vi "Set Cell Colors.vi"(0 "MulticolumnListbox in":refnum<vi>, 7 "Columns":T1[](array[typedef]), 9 "Table Items":string[][](array[string]), 11 "error in (no error)":errorcluster) -> (4 "MulticolumnListbox out":refnum<vi>, 15 "error out":errorcluster)   [LabVIEW 2015, in "KTable.xctl"]
uses:
  KTable.xctl
  ColumnSpec.ctl
  ColumnType.ctl
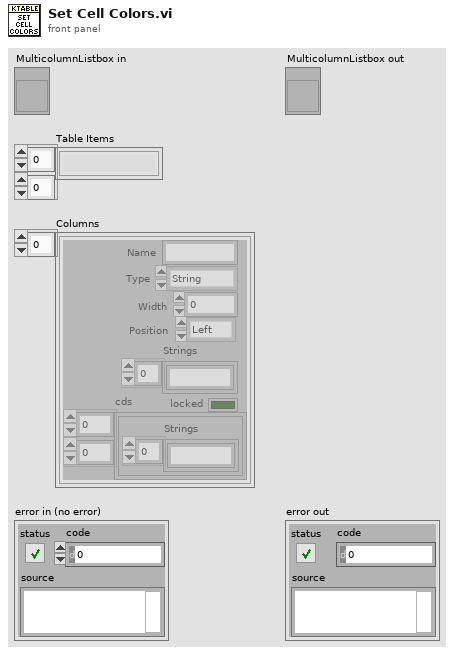
[diagram p1: front panel]
types:
  T1 = typedef "KTable.xctl/ColumnSpec.ctl" = cluster{"Name":string, "Type":T2, "Width":i32, "Strings":string[], "Position":enum16{"Left", "Center", "Right"}, "locked":bool, "cds":cluster{"Strings":string[]}[][]}
  T2 = typedef "KTable.xctl/ColumnType.ctl" = enum16{"String", "Enum", "Int", "Double", "Boolean", "Ring", "Formula", "Color"}
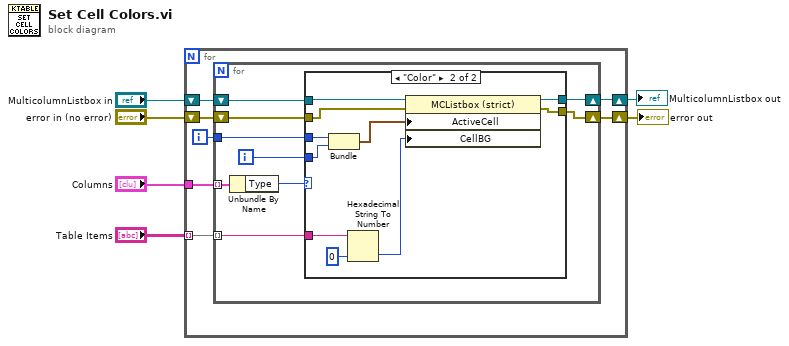
[diagram p0: block diagram]
diagram:
  n1 = for {
    tunnel: "Table Items" -> [w13] mode=indexing
    tunnel: "Columns" -> [w12]
    shift-right: [w9] -> w2
    shift-left: "MulticolumnListbox in" -> [w11]
    shift-right: [w8] -> w1
    shift-left: "error in (no error)" -> [w10]
    i -> [w7]
    n2 = for {
      tunnel: w13 -> [w14] mode=indexing
      tunnel: w12 -> [w22] mode=indexing
      shift-right: [w18] -> w9
      shift-left: w11 -> [w20]
      shift-right: [w17] -> w8
      shift-left: w10 -> [w19]
      tunnel: w7 -> [w16]
      i -> [w15]
      n3 = Unbundle By Name(w22) -> ("Type"=w21:T2)
      n4 = case shown="\"Color\"" w21 {
        tunnel: w20 -> [w24 w34]
        tunnel: w19 -> [w23 w33]
        tunnel: [w24 w32] -> w18
        tunnel: [w23 w31] -> w17
        tunnel: w16 -> [_ w30]
        tunnel: w15 -> [_ w29]
        tunnel: w14 -> [_ w27]
        frame "String", Default {
        }
        frame "Color" {
          n5 = Bundle(w30, w29) -> (w28:cluster{i32, i32})  [unwired: 1 in]
          n6 = Hexadecimal String To Number(string=w27, default (0uL)=u32 0 ("default (0 U32)")) -> (number=w26:u32)  [unwired: 1 in, 1 out]
          n7 = property class="MCListbox (strict)"(reference=w34, error in=w33, "ActiveCell"=w28, "CellBG"=w26) -> (reference out=w32:refnum<vi>, error out=w31:errorcluster)
        }
      }
    }
  }
  "error out" <- w1
  "MulticolumnListbox out" <- w2
